vi "TCP_Client.vi"() -> ()   [LabVIEW 2023]
panel:
  out "压力图":i32(graph)
  out "Weight/g":dbl
  in  "Ñ¡ÔñÎÄ¼þ´æ´¢Î»ÖÃÃ":path
  out "服务器端口号":dbl=8086.0
  out "服务器IP":string="192.168.4.1"
  out "湿度":dbl
  out "温度":dbl
  in  "设置采样间隔":dbl
  out "湿度图":dbl(graph)
  out "温度图":dbl(graph)
  out "湿度计":dbl(slide) scale=10.0..100.0
  out "温度计":dbl(slide) scale=10.0..60.0
  in  "停止按钮":bool
  in  "发送指令确认按键":bool
  in  "停止":bool
  # "TCP_Client"
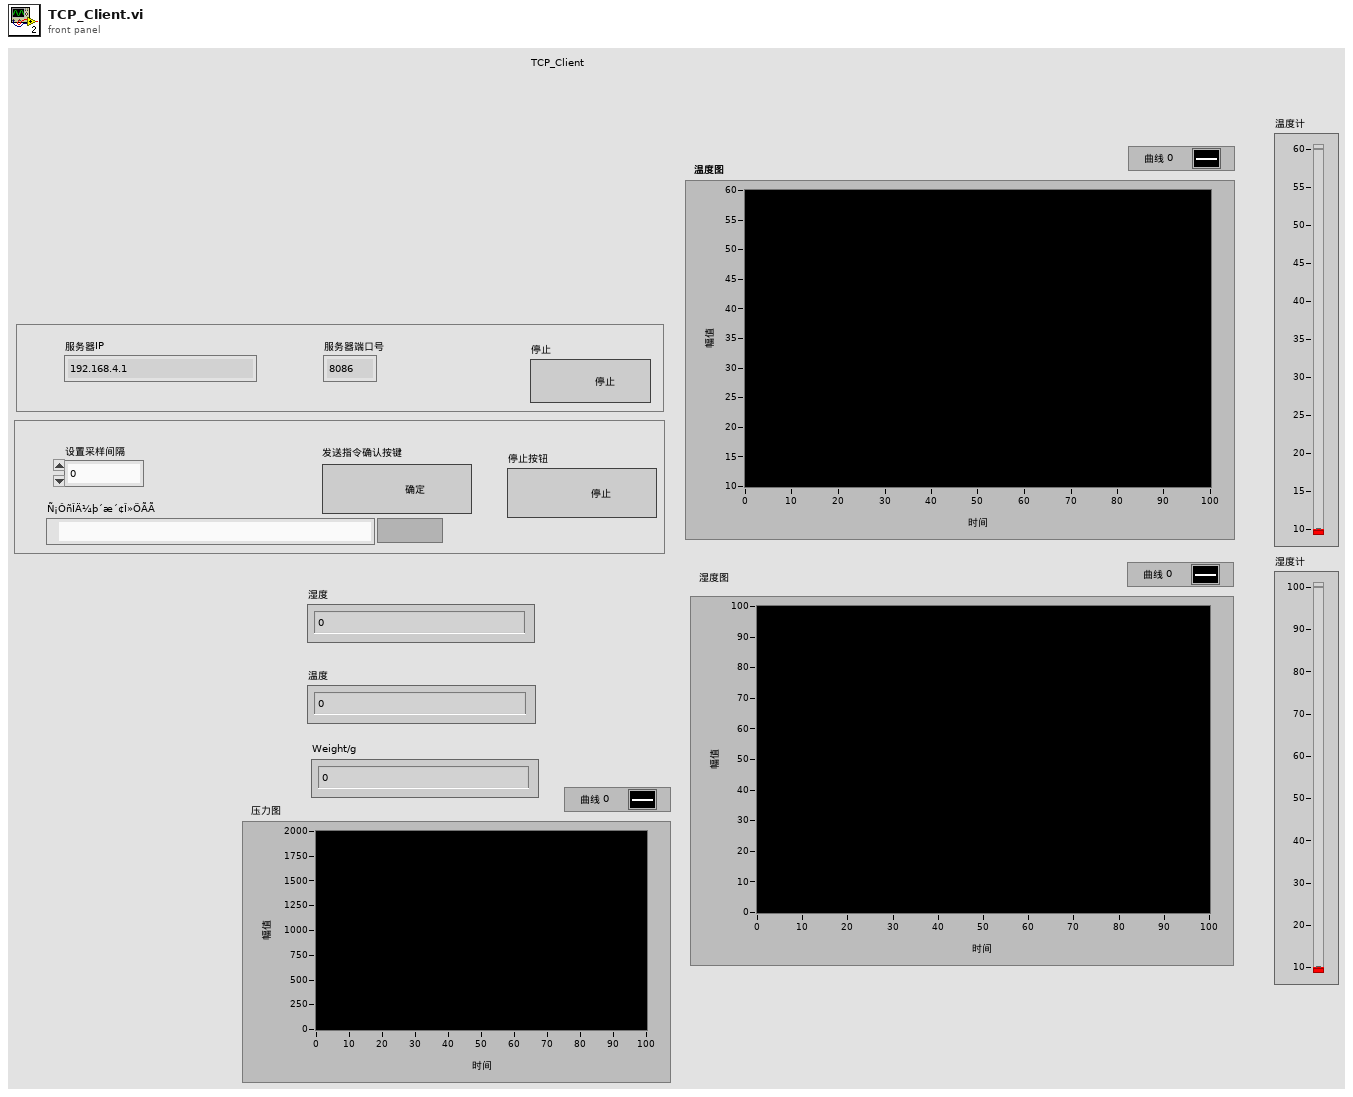
[diagram p1: front panel]
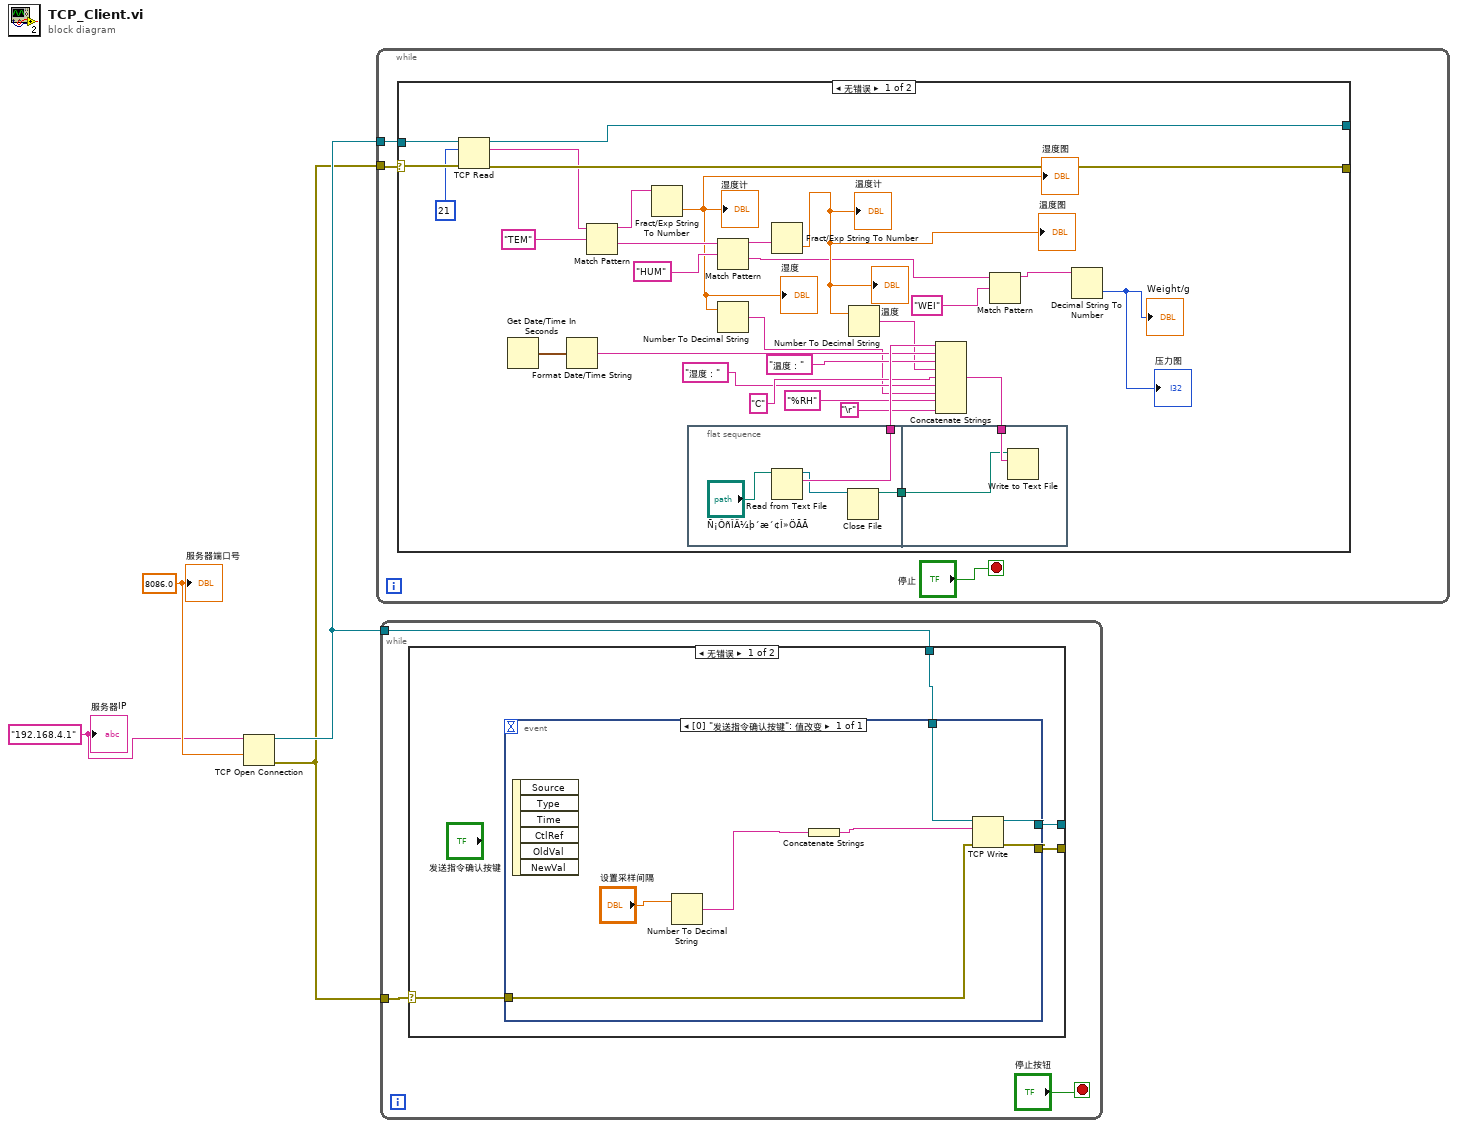
[diagram p0: block diagram]
diagram:
  w4 = 8086.0 ("服务器端口号")
  w1 = "192.168.4.1" ("服务器IP")
  n1 = TCP Open Connection(address=w1, remote port or service name=w4) -> (connection ID=w3:refnum<k5>, error out=w2:errorcluster)  [unwired: 3 in]
  n2 = while {
    tunnel: w2 -> [w7]
    tunnel: w3 -> [w6]
    stop <- "停止" stop-if-true
    n3 = case shown="无错误" w7 {
      selector: w7 -> [w32 w43]
      tunnel: w6 -> [w33 w44]
      tunnel: [w35 w43] -> _
      tunnel: [w34 w44] -> _
      frame No Error {
        n4 = TCP Read(connection ID=w33, bytes to read=21, error in (no error)=w32) -> (connection ID out=w34:refnum<k5>, data out=w27:string, error out=w35:errorcluster)  [unwired: 2 in]
        n5 = Get Date/Time In Seconds() -> (seconds since 1Jan1904=w23:timestamp)
        n6 = Format Date/Time String(seconds (now)=w23) -> (date/time string=w21:string)  [unwired: 2 in]
        n7 = Match Pattern(string=w27, regular expression="TEM") -> (before substring=w28:string, after substring=w31:string)  [unwired: 1 in, 2 out]
        n8 = Fract/Exp String To Number(string=w28) -> (number=w18:dbl)  [unwired: 3 in, 1 out]
        "湿度计" <- w18
        "湿度图" <- w18
        "湿度" <- w18
        n9 = flat-sequence {
          tunnel: [w39] -> w26
          tunnel: [w37] -> w24
          tunnel: w25 -> [w42]
          tunnel: w24 -> [w41]
          frame #0 {
            n10 = Read from Text File(file (use dialog)="Ñ¡ÔñÎÄ¼þ´æ´¢Î»ÖÃÃ") -> (refnum out=w38:refnum<file>, text=w39:string)  [unwired: 3 in, 2 out]
            n11 = Close File(refnum=w38) -> (path=w37:path)  [unwired: 1 in, 1 out]
          }
          frame #1 {
            n12 = Write to Text File(file (use dialog)=w41, text=w42) -> ()  [unwired: 2 in, 3 out]
          }
        }
        n13 = Match Pattern(string=w31, regular expression="HUM") -> (before substring=w22:string, after substring=w11:string)  [unwired: 1 in, 2 out]
        n14 = Number To Decimal String(number=w18) -> (decimal integer string=w15:string)  [unwired: 1 in]
        n15 = Fract/Exp String To Number(string=w22) -> (number=w12:dbl)  [unwired: 3 in, 1 out]
        "温度计" <- w12
        "温度图" <- w12
        "温度" <- w12
        n16 = Number To Decimal String(number=w12) -> (decimal integer string=w19:string)  [unwired: 1 in]
        n17 = Concatenate Strings(w26, w21, "温度：", w19, "C", "湿度：", w15, "%RH", "\r") -> (w25:string)
        n18 = Match Pattern(string=w11, regular expression="WEI") -> (before substring=w9:string)  [unwired: 1 in, 3 out]
        n19 = Decimal String To Number(string=w9) -> (number=→"Weight/g" →"压力图":i32)  [unwired: 2 in, 1 out]
      }
      frame Error {
      }
    }
  }
  n20 = while {
    tunnel: w2 -> [w47]
    tunnel: w3 -> [w46]
    stop <- "停止按钮" stop-if-true
    n21 = case shown="无错误" w47 {
      selector: w47 -> [w51 w60]
      tunnel: w46 -> [w50 w59]
      tunnel: [w49 w60] -> _
      tunnel: [w48 w59] -> _
      frame No Error {
        n22 = event shown="[0] \"发送指令确认按键\": 值改变" {
          selector: _ -> [_]
          dyn-events: _ -> [_]
          timeout: _ -> [_]
          tunnel: w51 -> [w54]
          tunnel: w50 -> [w55]
          tunnel: [w58] -> w49
          tunnel: [w57] -> w48
          event "发送指令确认按键": Value Change {
            n23 = event-data() -> ()  [unwired: 1 in, 6 out]
            n24 = Number To Decimal String(number="设置采样间隔") -> (decimal integer string=w52:string)  [unwired: 1 in]
            n25 = Concatenate Strings(w52) -> (w56:string)
            n26 = TCP Write(connection ID=w55, data in=w56, error in (no error)=w54) -> (connection ID out=w57:refnum<k5>, error out=w58:errorcluster)  [unwired: 1 in, 1 out]
          }
        }
      }
      frame Error {
      }
    }
  }
  "服务器IP" <- w1
  "服务器端口号" <- w4
